vi "EX 9-3 Blink MouseClick.vi"() -> ()   [LabVIEW 2011]
uses:
  <vilib>/LabVIEW Interface for Arduino/Type Defs/Board Type.ctl
  <vilib>/LabVIEW Interface for Arduino/Type Defs/Connection Type.ctl
  <vilib>/LabVIEW Interface for Arduino/Type Defs/Pin Mode.ctl
  <vilib>/Utility/inputDevices.llb/closeMouse.vi
  <vilib>/Utility/inputDevices.llb/mouseAcquire.vi
  <vilib>/LabVIEW Interface for Arduino/LabVIEW Interface for Arduino.lvlib
panel:
  out "button info":T1
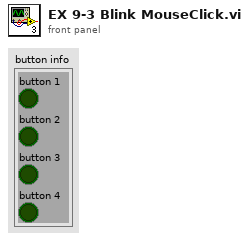
[diagram p1: front panel]
types:
  T1 = cluster{"button 1":bool, "button 2":bool, "button 3":bool, "button 4":bool}
  T2 = typedef "LabVIEW Interface for Arduino.lvlib/Pin Mode.ctl" = enum8{"Input", "Output"}
  T3 = typedef "LabVIEW Interface for Arduino.lvlib/Connection Type.ctl" = enum8{"USB / Serial", "XBEE", "BlueSmirf (Bluetooth)"}
  T4 = typedef "LabVIEW Interface for Arduino.lvlib/Board Type.ctl" = enum16{"Uno", "Dimuelanove w/Atmega 328", "Mega 2560"}
  T5 = typedef "LabVIEW Interface for Arduino.lvlib/Arduino Resource.ctl" = cluster{"VISA resource":refnum<visa-resource-name>, "Board Type":T4, "Connection Type":enum8{"USB / Serial"}, "Bytes Per Packet (15)":u8}
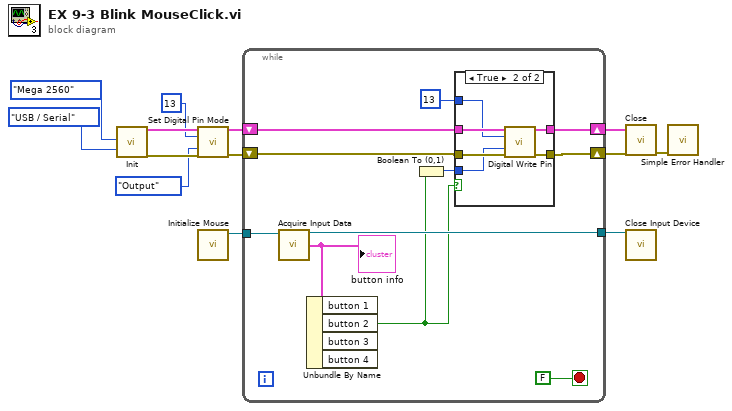
[diagram p0: block diagram]
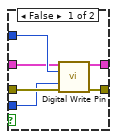
[diagram p2: hidden frame]
diagram:
  n1 = call <vilib>:"Init.vi"("Board Type (Uno)"=Board_Type."Mega 2560", "Connection Type (USB/Serial)"=Connection_Type."USB / Serial") -> ("Arduino Resource"=w6:T5, "error out"=w3:errorcluster)  [unwired: 16 in]
  n2 = call <vilib>:"Set Digital Pin Mode.vi"("Arduino Resource"=w6, "Digital I/O Pin"=u8 13, "Pin Mode (Input)"=Pin_Mode."Output", "error in"=w3) -> ("Arduino Resource"=w5:T5, "error out"=w4:errorcluster)  [unwired: 10 in]
  n3 = call <vilib>:"Initialize Mouse.vi"() -> ("device ID"=w8:refnum<k1>)  [unwired: 10 in, 1 out]
  n4 = while {
    shift-right: [w23] -> w13
    shift-left: w5 -> [w16]
    shift-right: [w22] -> w12
    shift-left: w4 -> [w15]
    tunnel: w8 -> [w21]
    tunnel: [w20] -> w7
    stop <- FALSE stop-if-true
    n5 = call-poly <vilib>:"Acquire Input Data.vi"("device ID"=w21) -> ("device ID"=w20:refnum<k1>, "button info"=w19:T1)  [unwired: 15 in, 2 out]
    "button info" <- w19
    n6 = Unbundle By Name(w19) -> ("button 2"=w17:bool)  [unwired: 3 out]
    n7 = Boolean To (0,1)(Boolean=w17) -> (0, 1=w18:i16)
    n8 = case shown="True" w17 {
      tunnel: w16 -> [w28 w36]
      tunnel: [w27 w35] -> w23
      tunnel: [w26 w34] -> w22
      tunnel: w15 -> [w30 w33]
      tunnel: u8 13 ("Digital I/O Pin") -> [w29 w32]
      tunnel: w18 -> [w25 w31]
      frame False {
        n9 = call <vilib>:"Digital Write Pin.vi"("Arduino Resource"=w28, "Digital I/O Pin (0)"=w29, "Value (0)"=w25, "error in"=w30) -> ("Arduino Resource"=w27:T5, "error out"=w26:errorcluster)  [unwired: 10 in]
      }
      frame True {
        n10 = call <vilib>:"Digital Write Pin.vi"("Arduino Resource"=w36, "Digital I/O Pin (0)"=w32, "Value (0)"=w31, "error in"=w33) -> ("Arduino Resource"=w35:T5, "error out"=w34:errorcluster)  [unwired: 10 in]
      }
    }
  }
  n11 = call <vilib>:"Close.vi"("Arduino Resource"=w13, "error in"=w12) -> ("error out"=w11:errorcluster)  [unwired: 13 in]
  n12 = call-poly <vilib>:"Close Input Device.vi"("device ID"=w7) -> ()  [unwired: 9 in, 1 out]
  n13 = call <vilib>:"Simple Error Handler.vi"("error in (no error)"=w11) -> ()  [unwired: 4 in, 5 out]
